vi "new.vi"(6 "stopTimeout[ms]":i32=5000, 8 "error in (no error)":errorcluster, 11 "task":refnum<class "ITask.lvclass">) -> (0 "error out":errorcluster, 3 "TaskController out":refnum<class "TaskController.lvclass">)   [LabVIEW 2023, in "TLC_Daemon.lvlib" / "TaskController.lvclass"]
doc: "Constructor\nNote: TaskController handles the life cycle of a single task.\nUse more TaskController objects if you want to handle more tasks.\n_____________________________________\nTLC Daemon 1.0.0.2\nCopyright (c) 2026 Andrea Cadei"
uses:
  TaskController.lvclass
  ITask/ITask.lvclass
  status.ctl
  TaskController.lvclass/TaskController.ctl
  ITaskStopMechanism/ITaskStopMechanism.lvclass
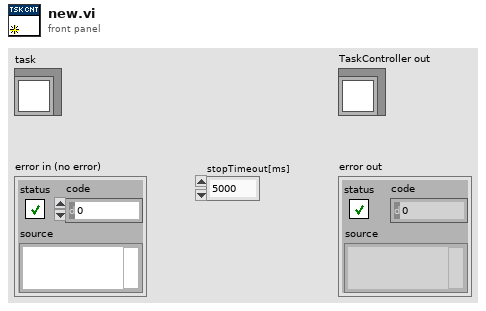
[diagram p1: front panel]
types:
  T1 = typedef "TLC_Daemon.lvlib/TaskController.lvclass/status.ctl" = enum16{"NotReady", "Ready", "Running", "Stopped", "Unknown"}
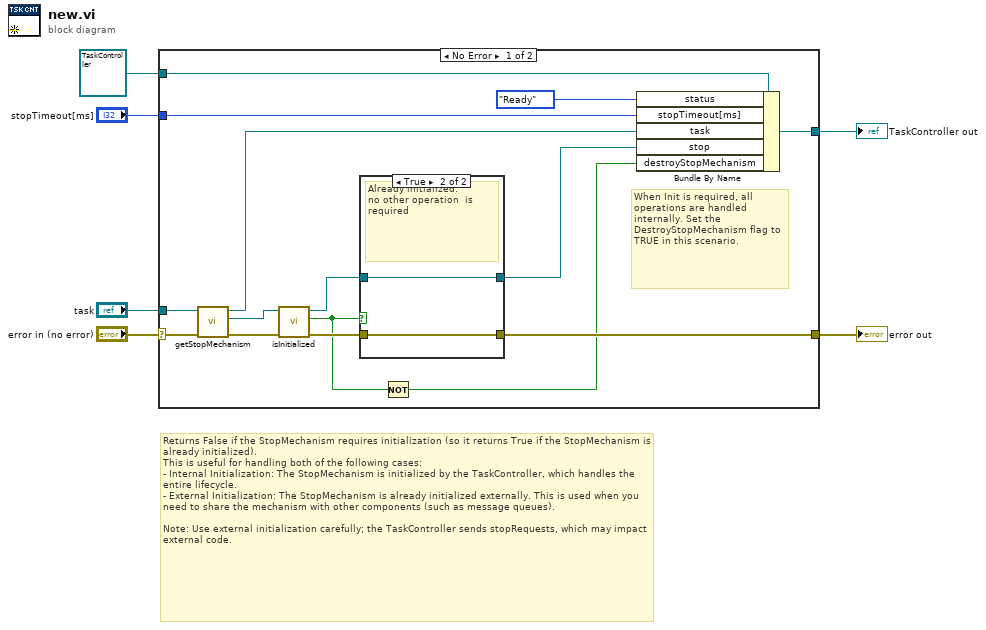
[diagram p0: block diagram]
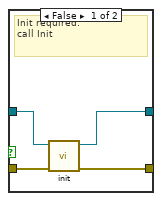
[diagram p2: hidden frame]
diagram:
  # "Returns False if the StopMechanism requires initialization (so it returns True if the StopMechanism is already initialized).\nThis is useful for handling both of the following cases:\n- Internal Initialization: The StopMechanism is initialized by the TaskController, which handles the entire lifecycle.\n- External Initialization: The StopMechanism is already initialized externally. This is used when you need to share the mechanism with other components (such as message queues).\n\nNote: Use external initialization carefully; the TaskController sends stopRequests, which may impact external code."
  n1 = case shown="No Error" "error in (no error)" {
    selector: "error in (no error)" -> [w19 w29]
    tunnel: [w11 w29] -> w5
    tunnel: [w20 w28] -> w3
    tunnel: refnum<class "TaskController.lvclass"> refnum ("TaskController in") -> [w21 w28]
    tunnel: "task" -> [w17 _]
    tunnel: "stopTimeout[ms]" -> [w9 _]
    frame No Error {
      # "When Init is required, all operations are handled internally. Set the DestroyStopMechanism flag to TRUE in this scenario."
      n2 = call-dynamic "getStopMechanism.vi"("error in (no error)"=w19, "ITask in"=w17) -> ("error out"=w16:errorcluster, "stopMechanism"=w13:refnum<class "ITaskStopMechanism.lvclass">, "ITask out"=w18:refnum<class "ITask.lvclass">)  [unwired: 7 in]
      n3 = call-dynamic "isInitialized.vi"("error in (no error)"=w16, "ITaskStopMechanism in"=w13) -> ("error out"=w14:errorcluster, "isInitRequired"=w8:bool, "ITaskStopMechanism out"=w15:refnum<class "ITaskStopMechanism.lvclass">)  [unwired: 7 in]
      n4 = case shown="True" w8 {
        tunnel: w15 -> [w24 w26]
        tunnel: w14 -> [w25 w27]
        tunnel: [w23 w26] -> w12
        tunnel: [w22 w27] -> w11
        frame False {
          # "Init required:\ncall Init"
          n5 = call-dynamic "init.vi"("error in (no error)"=w25, "ITaskStopMechanism in"=w24) -> ("error out"=w22:errorcluster, "ITaskStopMechanism out"=w23:refnum<class "ITaskStopMechanism.lvclass">)  [unwired: 8 in]
        }
        frame True {
          # "Already initialized:\nno other operation  is required"
        }
      }
      n6 = Not(x=w8) -> (.not. x?=w7:bool)
      n7 = Bundle By Name(cluster=w21, "status"=status."Ready", "stopTimeout[ms]"=w9, "task"=w18, "stop"=w12, "destroyStopMechanism"=w7) -> (w20:refnum<class "TaskController.lvclass">)
    }
    frame Error {
    }
  }
  "error out" <- w5
  "TaskController out" <- w3
